vi "ChooseOffensivePlay.vi"(8 "error in (no error)":errorcluster, 11 "Playbook_v2 in":refnum<class "Playbook_v2.lvclass">) -> (0 "error out":errorcluster, 3 "Playbook_v2 out":refnum<class "Playbook_v2.lvclass">)   [LabVIEW 2023, in "Playbook_v2.lvclass"]
uses:
  Playbook_v2.lvclass
  NewPlays/Play_v2_class/Play_v2.lvclass
  Playbook_v2.lvclass/Playbook_v2.ctl
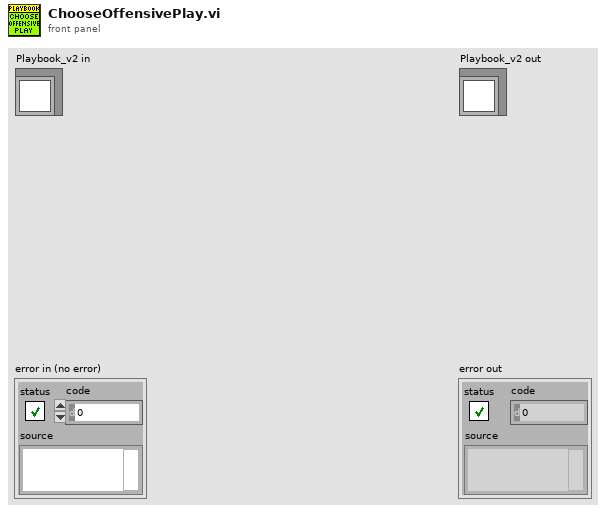
[diagram p1: front panel]
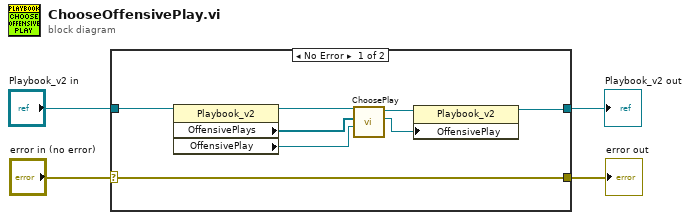
[diagram p0: block diagram]
diagram:
  n1 = case shown="No Error" "error in (no error)" {
    selector: "error in (no error)" -> [w12 w14]
    tunnel: [w12 w14] -> w3
    tunnel: [w5 w13] -> w1
    tunnel: "Playbook_v2 in" -> [w11 w13]
    frame No Error {
      n2 = property class="Playbook_v2"(reference=w11) -> (reference out=w10:refnum<class "Playbook_v2.lvclass">, "OffensivePlays"=w9:refnum<class "Play_v2.lvclass">[], "OffensivePlay"=w8:refnum<class "Play_v2.lvclass">)  [unwired: 1 in, 1 out]
      n3 = call "ChoosePlay.vi"("currentPlay"=w8, "plays"=w9, "Playbook_v2 in"=w10) -> ("newPlay"=w6:refnum<class "Play_v2.lvclass">, "Playbook_v2 out"=w7:refnum<class "Playbook_v2.lvclass">)  [unwired: 6 in, 1 out]
      n4 = property class="Playbook_v2"(reference=w7, "OffensivePlay"=w6) -> (reference out=w5:refnum<class "Playbook_v2.lvclass">)  [unwired: 1 in, 1 out]
    }
    frame Error {
    }
  }
  "error out" <- w3
  "Playbook_v2 out" <- w1
